vi "write_global_from_config_file.vi"   [LabVIEW 2011]
uses:
  global.vi
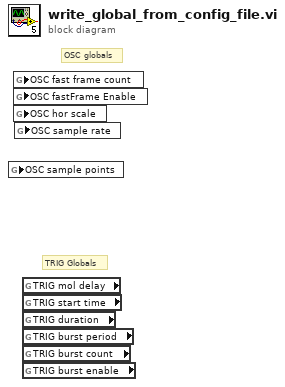
[diagram p0: block diagram]
diagram:
  # "TRIG Globals"
  # "OSC globals"
  n1 = global read "global.vi" "OSC sample points"() -> ()  [unwired: 1 in]
  n2 = global read "global.vi" "OSC fast frame count"() -> ()  [unwired: 1 in]
  n3 = global read "global.vi" "OSC fastFrame Enable"() -> ()  [unwired: 1 in]
  n4 = global read "global.vi" "OSC hor scale"() -> ()  [unwired: 1 in]
  n5 = global read "global.vi" "OSC sample rate"() -> ()  [unwired: 1 in]
  n6 = global read "global.vi" "TRIG mol delay"() -> (w1:dbl)
  n7 = global read "global.vi" "TRIG start time"() -> (w4:dbl[])
  n8 = global read "global.vi" "TRIG duration"() -> (w3:dbl[])
  n9 = global read "global.vi" "TRIG burst period"() -> (w2:dbl)
  n10 = global read "global.vi" "TRIG burst count"() -> ()  [unwired: 1 out]
  n11 = global read "global.vi" "TRIG burst enable"() -> ()  [unwired: 1 out]
